vi "queue_array_front.vi"(8 "error in":errorcluster, 10 "array":string[](array[string])=["Data: Initialize", "Initialize Core Data", "Data: Get Case Strings", "Data: Get Case Documentation", "UI: Initialize", "UI: Front Panel State >> Open", "Delay >> 1000"], 11 "queue in":refnum<queue>) -> (0 "error out":errorcluster, 3 "queue out":refnum<queue>)   [LabVIEW 2012]
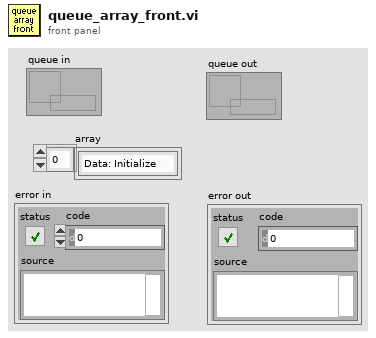
[diagram p1: front panel]
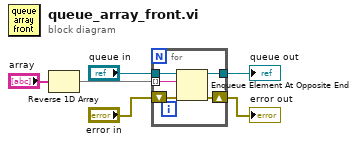
[diagram p0: block diagram]
diagram:
  n1 = Reverse 1D Array(array="array") -> (reversed array=w6:string[])
  n2 = for {
    tunnel: [w11] -> w5
    tunnel: "queue in" -> [w10]
    shift-right: [w8] -> w4
    shift-left: "error in" -> [w9]
    tunnel: w6 -> [w7] mode=indexing
    n3 = Enqueue Element At Opposite End(queue=w10, element=w7, error in (no error)=w9) -> (queue out=w11:refnum<queue>, error out=w8:errorcluster)  [unwired: 1 in, 1 out]
  }
  "queue out" <- w5
  "error out" <- w4
